vi "Load Device Config.vi"(8 "Error In":errorcluster, 11 "LINX Device Config":T1) -> (0 "Error Out":errorcluster, 3 "LINX Device Config":T1)   [LabVIEW 2020, in "Device.lvlib"]
uses:
  Device.lvlib
  Type Defs/LINX Device Config.ctl
  Type Defs/Interface.ctl
  Type Defs/TCP Config.ctl
  Type Defs/Channels.ctl
  LMH-LINX.lvlib
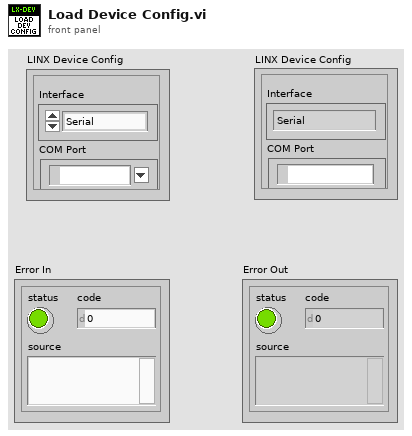
[diagram p1: front panel]
types:
  T1 = typedef "Device.lvlib/LINX Device Config.ctl" = cluster{"Interface":T2, "COM Port":refnum<visa-resource-name>, "TCP Configuration":T3, "Device Family":u8, "Device ID":u8, "Device Name":string, "TCP Ref":refnum<k5>, "Channels":T4}
  T2 = typedef "LMH-LINX.lvlib/Interface.ctl" = enum16{"Serial", "TCP"}
  T3 = typedef "Device.lvlib/TCP Config.ctl" = cluster{"IP Address":string, "Port":u16}
  T4 = typedef "LMH-LINX.lvlib/Channels.ctl" = cluster{"DI":u8[], "DO":u8[], "AI":u8[], "AO":u8[], "PWM":u8[], "QE":u8[], "UART":u8[], "I2C 2":u8[], "SPI":u8[], "CAN":u8[], "Servo":u8[], "AI Ref (V)":dbl, "AI Resolution (Bits)":u8, "AO Ref (V)":dbl, "AO Resolution (Bits)":u8}
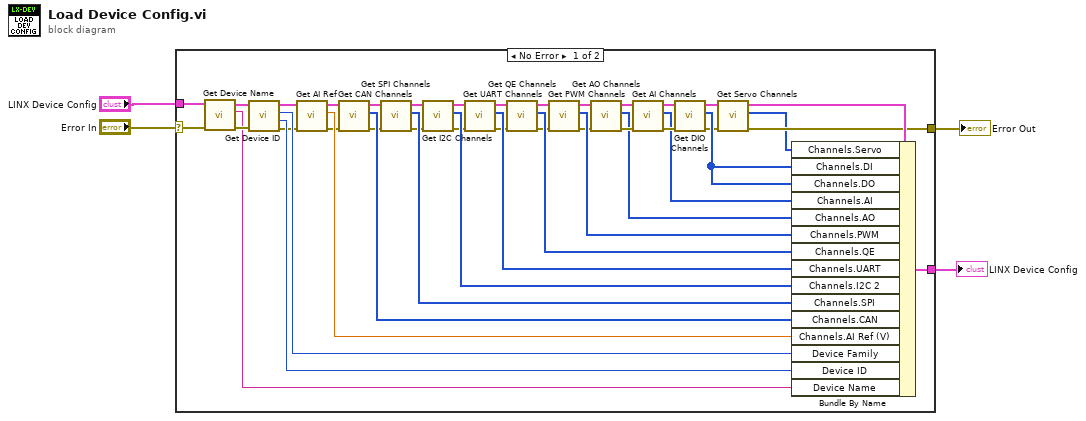
[diagram p0: block diagram]
diagram:
  n1 = case shown="No Error" "Error In" {
    selector: "Error In" -> [w5 w49]
    tunnel: [w15 w48] -> w4
    tunnel: "LINX Device Config" -> [w12 w48]
    tunnel: [w7 w49] -> w2
    frame No Error {
      n2 = call "Get Device Name.vi"("Error In"=w5, "LINX Device Config"=w12) -> ("Error Out"=w14:errorcluster, "Device Name"=w11:string, "LINX Device Config"=w13:T1)  [unwired: 7 in]
      n3 = call "Get Device ID.vi"("Error In"=w14, "LINX Device Config"=w13) -> ("Error Out"=w24:errorcluster, "Device ID"=w40:u8, "Device Family"=w39:u8, "LINX Device Config"=w23:T1)  [unwired: 6 in]
      n4 = call "Get AI Ref.vi"("Error In"=w24, "LINX Device Config"=w23) -> ("Error Out"=w25:errorcluster, "AI Ref"=w38:dbl, "LINX Device Config"=w22:T1)  [unwired: 7 in]
      n5 = call "Get CAN Channels.vi"("Error In"=w25, "LINX Device Config"=w22) -> ("Error Out"=w26:errorcluster, "CAN Channels"=w37:u8[], "LINX Device Config"=w21:T1)  [unwired: 6 in, 1 out]
      n6 = call "Get SPI Channels.vi"("Error In"=w26, "LINX Device Config"=w21) -> ("Error Out"=w27:errorcluster, "SPI Channels"=w36:u8[], "LINX Device Config"=w20:T1)  [unwired: 6 in, 1 out]
      n7 = call "Get I2C Channels.vi"("Error In"=w27, "LINX Device Config"=w20) -> ("Error Out"=w28:errorcluster, "I2C Channels"=w35:u8[], "LINX Device Config"=w19:T1)  [unwired: 6 in, 1 out]
      n8 = call "Get UART Channels.vi"("Error In"=w28, "LINX Device Config"=w19) -> ("Error Out"=w29:errorcluster, "UART Channels"=w34:u8[], "LINX Device Config"=w18:T1)  [unwired: 6 in, 1 out]
      n9 = call "Get QE Channels.vi"("Error In"=w29, "LINX Device Config"=w18) -> ("Error Out"=w30:errorcluster, "QE Channels"=w33:u8[], "LINX Device Config"=w17:T1)  [unwired: 6 in, 1 out]
      n10 = call "Get PWM Channels.vi"("Error In"=w30, "LINX Device Config"=w17) -> ("Error Out"=w31:errorcluster, "PWM Channels"=w32:u8[], "LINX Device Config"=w16:T1)  [unwired: 6 in, 1 out]
      n11 = call "Get AO Channels.vi"("Error In"=w31, "LINX Device Config"=w16) -> ("Error Out"=w47:errorcluster, "AI Channels"=w41:u8[], "LINX Device Config"=w45:T1)  [unwired: 6 in, 1 out]
      n12 = call "Get AI Channels.vi"("Error In"=w47, "LINX Device Config"=w45) -> ("Error Out"=w46:errorcluster, "AI Channels"=w42:u8[], "LINX Device Config"=w44:T1)  [unwired: 6 in, 1 out]
      n13 = call "Get DIO Channels.vi"("Error In"=w46, "LINX Device Config"=w44) -> ("Error Out"=w8:errorcluster, "DIO Channels"=w43:u8[], "LINX Device Config"=w10:T1)  [unwired: 6 in, 1 out]
      n14 = call "Get Servo Channels.vi"("Error In"=w8, "LINX Device Config"=w10) -> ("Error Out"=w7:errorcluster, "Servo Channels"=w6:u8[], "LINX Device Config"=w9:T1)  [unwired: 6 in, 1 out]
      n15 = Bundle By Name(cluster=w9, "Channels.Servo"=w6, "Channels.DI"=w43, "Channels.DO"=w43, "Channels.AI"=w42, "Channels.AO"=w41, "Channels.PWM"=w32, "Channels.QE"=w33, "Channels.UART"=w34, "Channels.I2C 2"=w35, "Channels.SPI"=w36, "Channels.CAN"=w37, "Channels.AI Ref (V)"=w38, "Device Family"=w39, "Device ID"=w40, "Device Name"=w11) -> (w15:T1)
    }
    frame Error {
    }
  }
  "Error Out" <- w2
  "LINX Device Config" <- w4
